vi "from string 1.0.vi"(8 "error in (no error)":errorcluster, 10 "data":string, 11 "Sequencer Module configuration in":refnum<class "Sequencer Module configuration.lvclass">) -> (0 "error out":errorcluster, 3 "Sequencer Module configuration out":refnum<class "Sequencer Module configuration.lvclass">)   [LabVIEW 2015, in "Sequencer Module configuration.lvclass"]
uses:
  Sequencer Module configuration.lvclass
  classes/Result Processor/Config/ResultProcessor Config.lvclass
  Line.ctl
  classes/Sequence/Config/Sequence Config.lvclass
  Sequencer Module configuration.lvclass/Sequencer Module configuration.ctl
  <vilib>/NI/Configuration Framework/serializable configuration/NISE_CEF_serializable configuration.lvclass
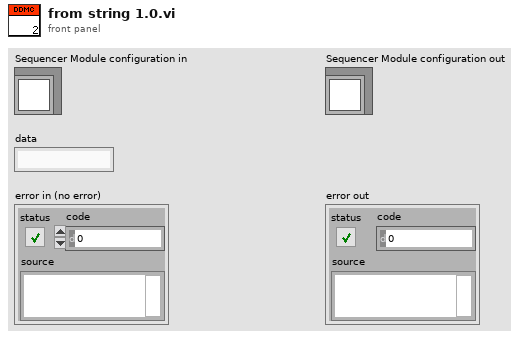
[diagram p1: front panel]
types:
  T1 = typedef "Sequencer Module configuration.lvclass/Line.ctl" = cluster{"Sequence":refnum<class "Sequence Config.lvclass">}
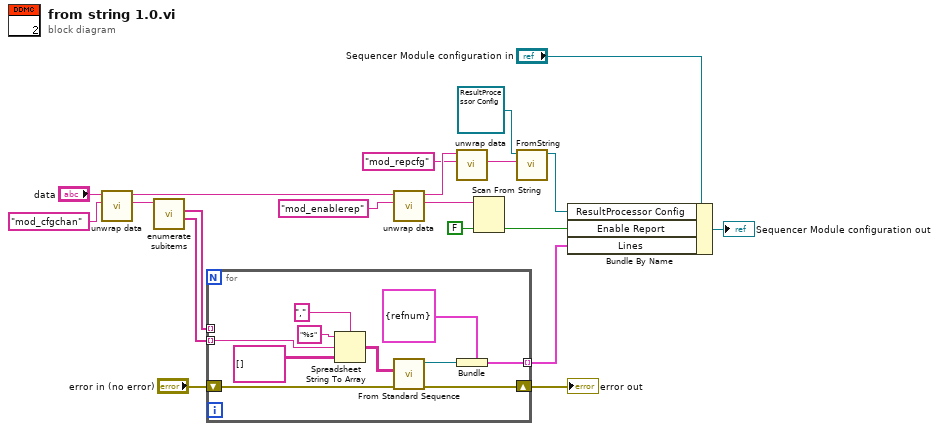
[diagram p0: block diagram]
diagram:
  n1 = call <vilib>:"unwrap data.vi"("identifier"="mod_cfgchan", "data to unwrap"="data") -> ("unwrapped data"=w15:string, "remaining string"=w10:string)  [unwired: 8 in]
  n2 = call <vilib>:"enumerate subitems.vi"("data to enumerate"=w15) -> ("associated data"=w14:string[], "discovered subitems"=w13:string[])  [unwired: 8 in, 1 out]
  n3 = for {
    shift-right: [w21] -> w20
    shift-left: "error in (no error)" -> [w22]
    tunnel: w13 -> [_] mode=indexing
    tunnel: w14 -> [w28] mode=indexing
    tunnel: [w29] -> w19 mode=indexing
    n4 = Spreadsheet String To Array(delimiter (Tab)=",", format string="%s", spreadsheet string=w28, array type (2D Dbl)=string[][] [] ("array")) -> (array=w25:string[][])
    n5 = call "From Standard Sequence.vi"("error in (no error)"=w22, "Standard Sequence"=w25) -> ("error out"=w21:errorcluster, "Sequence Config.lvclass"=w23:refnum<class "Sequence Config.lvclass">)  [unwired: 8 in]
    n6 = Bundle(cluster=T1 {"Sequence"=refnum} ("Line"), "Sequence"=w23) -> (w29:T1)
  }
  "error out" <- w20
  n7 = call <vilib>:"unwrap data.vi"("identifier"="mod_enablerep", "data to unwrap"=w10) -> ("unwrapped data"=w3:string, "remaining string"=w9:string)  [unwired: 8 in]
  n8 = call <vilib>:"unwrap data.vi"("identifier"="mod_repcfg", "data to unwrap"=w9) -> ("unwrapped data"=w6:string)  [unwired: 8 in, 1 out]
  n9 = Scan From String(input string=w3, default 1=FALSE ("Enable Report")) -> (output 1=w1:bool)  [unwired: 3 in, 3 out]
  n10 = call-dynamic "FromString.vi"("data"=w6, "ResultProcessor Config in"=refnum<class "ResultProcessor Config.lvclass"> refnum) -> ("ResultProcessor Config out"=w4:refnum<class "ResultProcessor Config.lvclass">)  [unwired: 8 in, 1 out]
  n11 = Bundle By Name(cluster="Sequencer Module configuration in", "ResultProcessor Config"=w4, "Enable Report"=w1, "Lines"=w19) -> (→"Sequencer Module configuration out":refnum<class "Sequencer Module configuration.lvclass">)
